vi "Test Mode Global.vi"() -> ()   [LabVIEW 2018]
panel:
  out "System Tests":T1
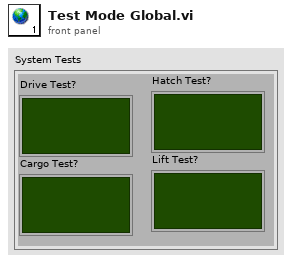
[diagram p1: front panel]
types:
  T1 = cluster{"Drive Test?":bool, "Cargo Test?":bool, "Hatch Test?":bool, "Lift Test?":bool}
diagram:
